vi "Group_ToClass.vi"(8 "error in (no error)":errorcluster, 11 "Item Ref in":T1 format="%.0x") -> (0 "error out":errorcluster, 2 "Channels":T1[](array[typedef]) format="%.0x", 3 "Group out":refnum<class "Group.lvclass">)   [LabVIEW 2024, in "Embedded TDMS Logger System Explorer.lvlib"]
doc: "Creates a group class from the VeriStand System Definition File Custom Device group defined by the item ref in."
uses:
  Embedded TDMS Logger System Explorer.lvlib
  <vilib>/NI VeriStand/Custom Device API/Custom Device Item Ref.ctl
  Shared/File Classes/Group/Group.lvclass
  Shared/File Classes/Meta Data.ctl
  <vilib>/NI VeriStand/Custom Device API/Get Item Property (Variant).vi
  <vilib>/NI VeriStand/Custom Device API/Custom Device API.lvlib
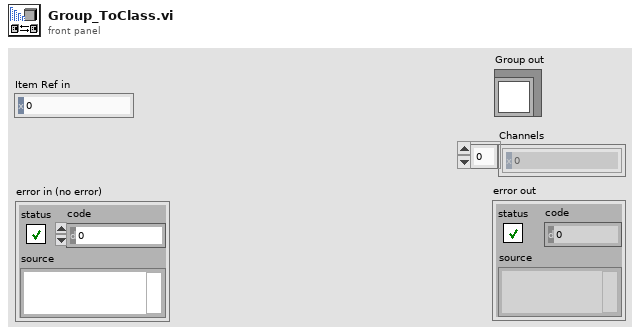
[diagram p1: front panel]
types:
  T1 = typedef "Custom Device API.lvlib/Custom Device Item Ref.ctl" = u64
  T2 = typedef "Meta Data.ctl" = cluster{"Key":string, "Value":string}
  T3 = typedef "Custom Device API.lvlib/Custom Device Item Info.ctl" = cluster{"Name":string, "Is Channel":bool, "GUID":string, "Is Waveform":bool}
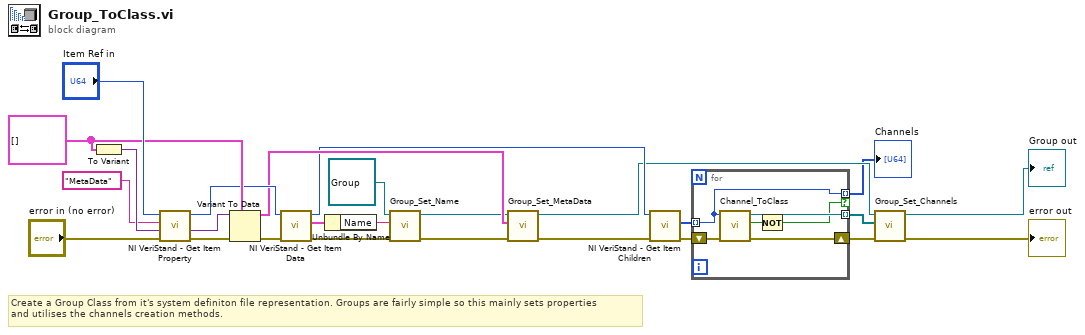
[diagram p0: block diagram]
diagram:
  w21 = T2[] []
  # "Create a Group Class from it's system definiton file representation. Groups are fairly simple so this mainly sets properties\nand utilises the channels creation methods."
  n1 = To Variant(anything=w21) -> (Variant=w26:variant)
  n2 = call-poly <vilib>:"NI VeriStand - Get Item Property.vi"("error in (no error)"="error in (no error)", "Default Value"=w26, "Property Name"="MetaData", "Item Ref in"="Item Ref in") -> ("error out"=w23:errorcluster, "Value"=w22:variant, "Item Ref out"=w20:T1)  [unwired: 4 in, 1 out]
  n3 = Variant To Data(error in=w23, type=w21, Variant=w22) -> (data=w13:T2[], error out=w19:errorcluster)
  n4 = call <vilib>:"NI VeriStand - Get Item Data.vi"("error in (no error)"=w19, "Item Ref in"=w20) -> ("error out"=w15:errorcluster, "Item Info"=w18:T3, "Item Ref out"=w10:T1)  [unwired: 7 out]
  n5 = Unbundle By Name(w18) -> ("Name"=w17:string)
  n6 = call-dynamic "Group_Set_Name.vi"("error in (no error)"=w15, "Name"=w17, "Group in"=refnum<class "Group.lvclass"> refnum ("Group.lvclass")) -> ("error out"=w14:errorcluster, "Group out"=w12:refnum<class "Group.lvclass">)  [unwired: 7 in]
  n7 = call-dynamic "Group_Set_MetaData.vi"("error in (no error)"=w14, "Meta Data"=w13, "Group in"=w12) -> ("error out"=w11:errorcluster, "Group out"=w7:refnum<class "Group.lvclass">)  [unwired: 7 in]
  n8 = call <vilib>:"NI VeriStand - Get Item Children.vi"("error in (no error)"=w11, "Item Ref in"=w10) -> ("error out"=w9:errorcluster, "Child Refs"=w8:T1[])  [unwired: 6 in, 2 out]
  n9 = for {
    shift-right: [w31] -> w5
    shift-left: w9 -> [w32]
    tunnel: w8 -> [w29] mode=indexing
    tunnel: [w30] -> w6 mode=indexing
    tunnel: [w29] -> w1 mode=indexing if=w27
    n10 = call "Channel_ToClass.vi"("error in (no error)"=w32, "Item Ref in"=w29) -> ("error out"=w31:errorcluster, "Wfm?"=w28:bool, "Channel out"=w30:refnum<class "Channel.lvclass">)  [unwired: 7 in]
    n11 = Not(x=w28) -> (.not. x?=w27:bool)
  }
  "Channels" <- w1
  n12 = call-dynamic "Group_Set_Channels.vi"("error in (no error)"=w5, "Channels"=w6, "Group in"=w7) -> ("error out"=→"error out":errorcluster, "Group out"=→"Group out":refnum<class "Group.lvclass">)  [unwired: 7 in]
